vi "Calibrate Gripper.vi"(2 "node":string, 3 "Side":T1, 6 "error in":errorcluster) -> (5 "error out":errorcluster)   [LabVIEW 2012]
doc: "Calibrate the left or right gripper"
uses:
  ROS/Code/SubVIs/_ROSDirection.ctl
  ROS/Code/Console/Servers/ServerSubs/TopicDef.ctl
  ROS/Code/SubVIs/BaxterSide.ctl
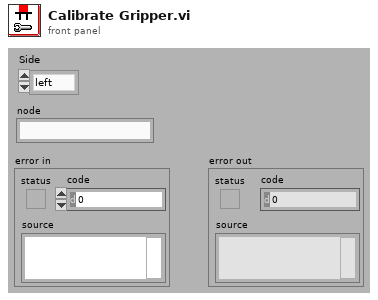
[diagram p1: front panel]
types:
  T1 = typedef "BaxterSide.ctl" = enum16{"left", "right"}
  T2 = typedef "TopicDef.ctl" = cluster{"Topic":string, "Type":string, "Action":T3, "Update (ms)":u16, "queue size":u16}
  T3 = typedef "_ROSDirection.ctl" = enum16{"Node", "Publisher", "Subscriber", "ServiceClient", "ServiceProvider"}
  T4 = enum16{"no_op", "set", "configure", "reboot", "reset", "calibrate", "clear_calibration", "prepare_to_grip", "grip", "release", "go", "stop"}
  T5 = typedef "_ROSControl.ctl" = cluster{"topic port":u16, "Node":string, "topic":string, "type":string, "node port":u16, "error ":errorcluster, "Direction":T3, "Update (ms)":u16, "FIFO size":u16}
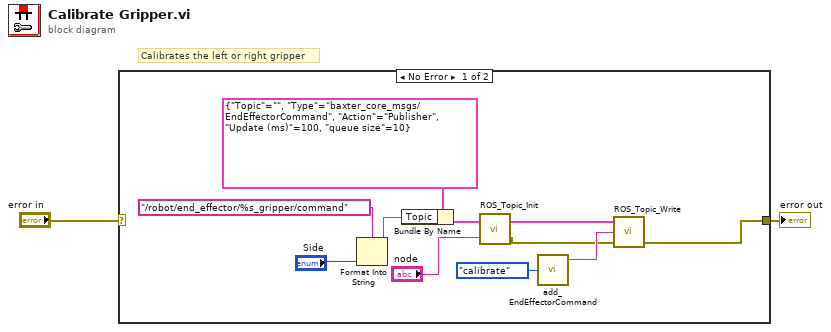
[diagram p0: block diagram]
diagram:
  # "Calibrates the left or right gripper"
  n1 = case shown="No Error" "error in" {
    selector: "error in" -> [_ w14]
    tunnel: [w4 w14] -> w2
    frame No Error {
      n2 = Format Into String(format string="/robot/end_effector/%s_gripper/command" ("Topic"), "Side") -> (resulting string=w9:string)  [unwired: 2 in, 1 out]
      n3 = Bundle By Name(cluster=T2 {"Topic"="", "Type"="baxter_core_msgs/EndEffectorCommand", "Action"=enum."Publisher", "Update (ms)"=100, "queue size"=10} ("Definitions"), "Topic"=w9) -> (w6:T2)
      n4 = call "ROS_Topic_Init.vi"("node"="node", "Definitions"=w6) -> ("error out"=w3:errorcluster, "ROS out"=w13:T5)
      n5 = call "add_EndEffectorCommand.vi"("Commands"=T4."calibrate") -> ("msg out"=w5:string)  [unwired: 4 in]
      n6 = call "ROS_Topic_Write.vi"("error in (no error)"=w3, "Msg in"=w5, "ROS in"=w13) -> ("error out"=w4:errorcluster)  [unwired: 1 in, 1 out]
    }
    frame Error {
    }
  }
  "error out" <- w2
